vi "sendValue.vi"(8 "error in (no error)":errorcluster, 10 "data":variant, 11 "exitControl in":refnum<class "exitControl.lvclass">) -> (0 "error out":errorcluster, 2 "function return":i32, 3 "exitControl out":refnum<class "exitControl.lvclass">)   [LabVIEW 2016, in "SALLV_AtDome_Messaging.lvlib" / "exitControl.lvclass"]
uses:
  exitControl.lvclass
  ts_sallv_AtDome/DataTypes/command_disable.ctl
  exitControl.lvclass/exitControl.ctl
  ts_sallv_AtDome/SALLV_AtDome.lvlib
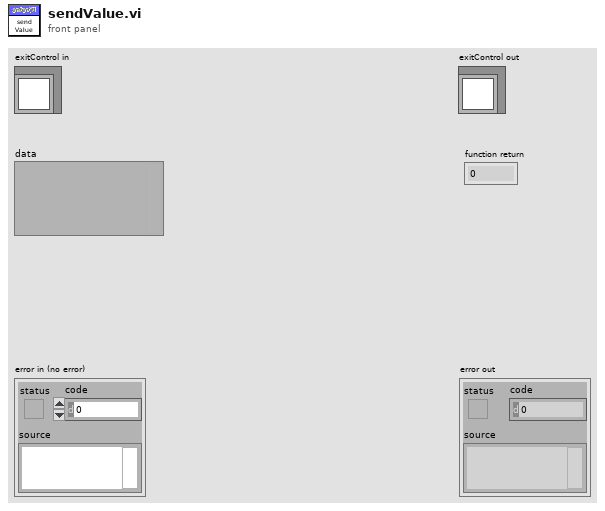
[diagram p1: front panel]
types:
  T1 = typedef "SALLV_AtDome_Messaging.lvlib/SALLV_AtDome.lvlib/command_disable.ctl" = cluster{"value":bool}
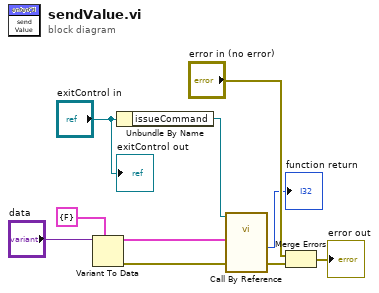
[diagram p0: block diagram]
diagram:
  n1 = Variant To Data(type=T1 {"value"=FALSE} ("command_exitControl_Ctl"), Variant="data") -> (data=w2:T1, error out=w1:errorcluster)  [unwired: 1 in]
  n2 = Unbundle By Name("exitControl in") -> ("issueCommand"=w7:refnum<vi>)
  n3 = call-by-ref "?"(reference=w7, "error in (no error)"=w1, "command_disable_Ctl"=w2) -> ("error out"=w8:errorcluster, "function return"=→"function return":i32)  [unwired: 8 in, 3 out]
  n4 = Merge Errors("error in (no error)", w8) -> (→"error out":errorcluster)
  "exitControl out" <- "exitControl in"
